vi "Get Parallel States.vi"(11 "Parallel Test in":refnum<class "Parallel Test.lvclass">) -> (2 "Positions":u32[][](array[numeric]), 3 "States":u32[](array[numeric]))   [LabVIEW 2015, in "Parallel Test.lvclass"]
doc: "This VI can be used as an override to modify the positions you're running within each parallel execution. The States output is used to define the state of each parallel loop. If all the positions in a loop are Failed and/or Idle you could set the the state to 'Failed'. To have the parallel test run set it to 'Running' The Positions output indicates which positions will run within that loops parallel execution. Do not include any previously Failed or Idle positions in a group set to Run. \n\nThe default behavior of this VI returns every available position with it's own current state. Do not override if you want to run a parallel loop for each of the UUTs."
uses:
  Parallel Test.lvclass
  Classes/Application/Class/Application.lvclass
  Test Class/Test Class.lvclass
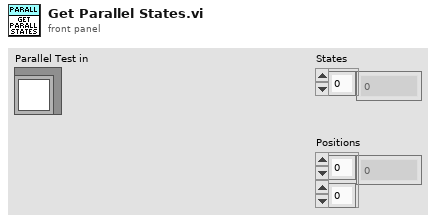
[diagram p1: front panel]
types:
  T1 = cluster{"Serial Number Reference":refnum<vi>, "Status Message Reference":refnum<vi>, "Position":u32}[]
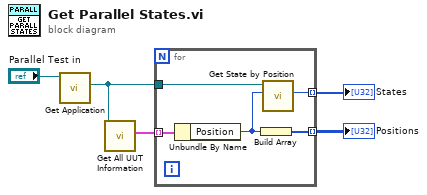
[diagram p0: block diagram]
diagram:
  n1 = call "Get Application.vi"("Test Class in"="Parallel Test in") -> ("Application.lvlib:Application.lvclass"=w3:refnum<class "Application.lvclass">)  [unwired: 9 in, 1 out]
  n2 = call-dynamic "Get All UUT Information.vi"("Application in"=w3) -> ("Active UUTs"=w4:T1)  [unwired: 8 in, 2 out]
  n3 = for {
    tunnel: w4 -> [w10] mode=indexing
    tunnel: w3 -> [w9]
    tunnel: [w8] -> w2 mode=indexing
    tunnel: [w6] -> w1 mode=indexing
    n4 = Unbundle By Name(w10) -> ("Position"=w7:u32)
    n5 = Build Array(w7) -> (w6:u32[])
    n6 = call-dynamic "Get State by Position.vi"("Position"=w7, "Application in"=w9) -> ("State"=w8:u32)  [unwired: 7 in, 2 out]
  }
  "States" <- w2
  "Positions" <- w1
